vi "WPI_DashboardEnsure File Extension.vi"(10 "Extension":string, 11 "Name":string) -> (3 "Name Out":string)   [LabVIEW 2025]
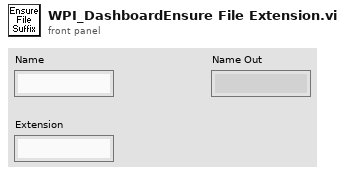
[diagram p1: front panel]
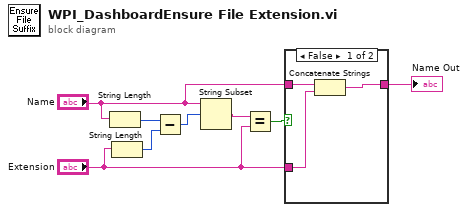
[diagram p0: block diagram]
diagram:
  n1 = String Length(string="Name") -> (length=w8:i32)
  n2 = String Length(string="Extension") -> (length=w7:i32)
  n3 = Subtract(x=w8, y=w7) -> (x-y=w6:i32)
  n4 = String Subset(string="Name", offset (0)=w6) -> (substring=w5:string)  [unwired: 1 in]
  n5 = Equal?(x=w5, y="Extension") -> (x = y?=w4:bool)
  n6 = case shown="False" w4 {
    tunnel: [w9 w12] -> w3
    tunnel: "Name" -> [w11 w12]
    tunnel: "Extension" -> [w10 _]
    frame False {
      n7 = Concatenate Strings(w11, w10) -> (w9:string)
    }
    frame True {
    }
  }
  "Name Out" <- w3
